vi "microphone.vi"   [LabVIEW 2018]
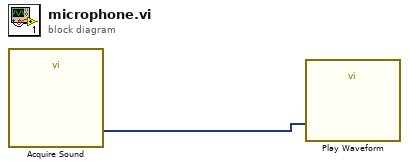
[diagram p0: block diagram]
diagram:
  n1 = call "Acquire Sound"() -> ("Data"=w1:dynamicdata)  [unwired: 18 in, 1 out]
  n2 = call "Play Waveform"("Data"=w1) -> ()  [unwired: 18 in, 1 out]
